vi "PNG&PIXMAP.vi"(6 "error in":errorcluster, 7 "Current png filename":string, 8 "Png path":path) -> (0 "error out":errorcluster, 2 "pixmap.bin":u32[](array[numeric]) format="%.0x", 3 "PNG Picture":picture)   [LabVIEW 2025]
panel:
  out "error out 2":errorcluster
  in  "error in 2":errorcluster
  out "Array 2D":u32[][](array[numeric]) format="%x"
  out "hauteur":u32
  out "largeur":u32
  out "image":u8[](array[numeric])
  out "image depth":i32
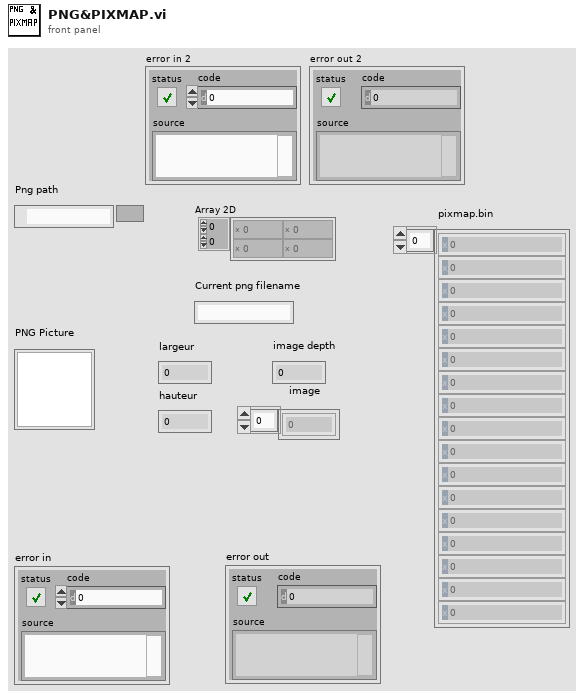
[diagram p1: front panel]
types:
  T1 = enum16{"open", "replace", "create", "open or create", "replace or create", "replace or create with confirmation"}
  T2 = enum16{"big-endian, network order", "native, host order", "little-endian"}
  T3 = typedef "imagedata.ctl" = cluster{"image type":i32, "image depth":i32, "image":u8[], "mask":u8[], "colors":u32[], "Rectangle":cluster{"left":i16, "top":i16, "right":i16, "bottom":i16}}
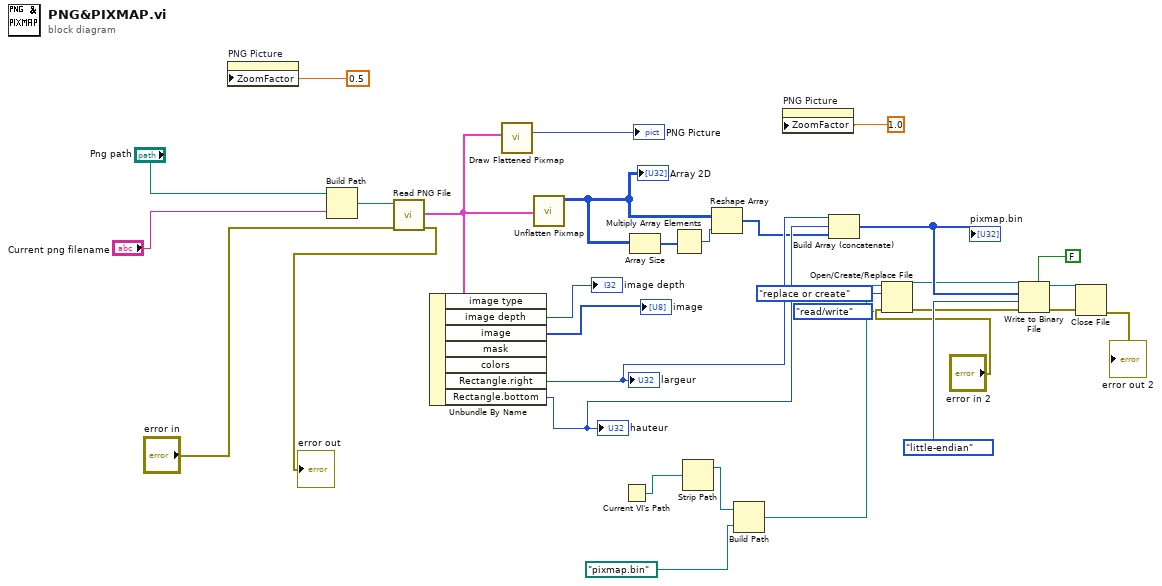
[diagram p0: block diagram]
diagram:
  n1 = property on="PNG Picture" class="Pict"("ZoomFactor"=0.5) -> ()  [unwired: 2 in, 2 out]
  n2 = Build Path(base path="Png path", name or relative path="Current png filename") -> (appended path=w15:path)
  n3 = call <vilib>:"Read PNG File.vi"("error in (no error)"="error in", "path to PNG file"=w15) -> ("error out"=→"error out":errorcluster, "image data"=w28:T3)  [unwired: 7 in, 1 out]
  n4 = Unbundle By Name(w28) -> ("image depth"=→"image depth":i32, "image"=→"image":u8[], "Rectangle.right"=w27:i16, "Rectangle.bottom"=w26:i16)  [unwired: 3 out]
  "largeur" <- w27
  "hauteur" <- w26
  n5 = call <vilib>:"Draw Flattened Pixmap.vi"("image data"=w28) -> ("new picture"=→"PNG Picture":picture)  [unwired: 8 in]
  n6 = call <vilib>:"Unflatten Pixmap.vi"("image data"=w28) -> ("24-bit pixmap"=w23:u32[][])  [unwired: 4 in, 6 out]
  "Array 2D" <- w23
  n7 = Current VI's Path() -> (path=w11:path)
  n8 = Array Size(array=w23) -> (size(s)=w25:i32[])
  n9 = Multiply Array Elements(1:w25) -> (0:w24:i32)
  n10 = Strip Path(path=w11) -> (stripped path=w10:path)  [unwired: 1 out]
  n11 = Reshape Array(w23, w24) -> (w22:u32[])
  n12 = Build Path(base path=w10, name or relative path=path "pixmap.bin") -> (appended path=w18:path)
  n13 = property on="PNG Picture" class="Pict"("ZoomFactor"=sgl 1.0 ("Zoom Factor")) -> ()  [unwired: 2 in, 2 out]
  n14 = Build Array (concatenate)(w27, w26, w22) -> (w21:u32[])
  "pixmap.bin" <- w21
  n15 = Open/Create/Replace File(file path (use dialog)=w18, error in="error in 2", operation (0:open)=T1."replace or create", access (0:read/write)=enum16{"read/write", "read-only", "write-only"}."read/write") -> (refnum out=w4:refnum<file>, error out=w6:errorcluster)  [unwired: 2 in, 1 out]
  n16 = Write to Binary File(file (use dialog)=w4, data=w21, error in=w6, 5:FALSE, 9:T2."little-endian" ("byte order (0:big-endian, network order)")) -> (refnum out=w8:refnum<file>, error out=w9:errorcluster)  [unwired: 1 in, 1 out]
  n17 = Close File(refnum=w8, error in=w9) -> (error out=→"error out 2":errorcluster)  [unwired: 1 out]
